vi "DecodeUInt64.vi"(1 "Data In":u8[](array[numeric])) -> (0 "Data Out":u64[](array[numeric]))   [LabVIEW 2014, in "navX Library v1 (deprecated).lvlib"]
uses:
  navX Library v1 (deprecated).lvlib
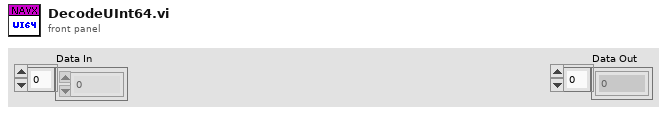
[diagram p1: front panel]
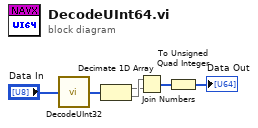
[diagram p0: block diagram]
diagram:
  n1 = call "DecodeUInt32.vi"("Data In"="Data In") -> ("Data Out"=w4:u32[])
  n2 = Decimate 1D Array(w4) -> (w5:u32[], w6:u32[])
  n3 = Join Numbers(hi=w6, lo=w5) -> ((hi.lo)=w2:u64[])
  n4 = To Unsigned Quad Integer(1:w2) -> (0:→"Data Out":u64[])
